vi "Teleop.vi"(10 "Match Info":T1={"Autonomous Elapsed Seconds"=0.0, "TeleOp Elapsed Seconds"=0.0, "Disabled Elapsed Seconds"=0.0, "Visited Autonomous"=FALSE, "Visited TeleOp"=FALSE, "Visited Disabled"=FALSE, "Autonomous Settings"={"Autonomous Style"=enum."Independent", "VI Refnum"=refnum}}, 11 "Call Context":T2) -> ()   [LabVIEW 2018]
doc: "This VI is called for each TeleOp packet received from the DS where the robot is not disabled. It is often used to read from the joysticks and update I/O or to update setpoints for timed control loops. It should complete and return within 20 milliseconds or it may miss DS packets."
uses:
  <vilib>/Rock Robotics/WPI/DriverStation/WPI_DriverStationDerivedRobotMode.ctl
  <vilib>/Rock Robotics/WPI/DriverStation/WPI_DriverStationMatch Info.ctl
  <vilib>/Rock Robotics/WPI/Solenoid/WPI_SolenoidValue.ctl
  <vilib>/Rock Robotics/WPI/Utilities/WPI_GetSetVariantRefNum.vi
  Robot Global Data.vi
  <vilib>/Rock Robotics/Network Tables/NT Write Numeric Array.vi
  <vilib>/Rock Robotics/WPI/Solenoid/WPI_SolenoidSetEnum.vi
  <vilib>/Rock Robotics/Network Tables/NT Write Number.vi
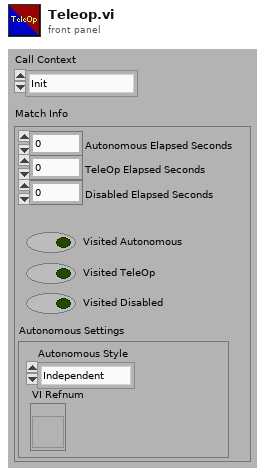
[diagram p1: front panel]
types:
  T1 = typedef "WPI_DriverStationMatch Info.ctl" = cluster{"Autonomous Elapsed Seconds":dbl, "TeleOp Elapsed Seconds":dbl, "Disabled Elapsed Seconds":dbl, "Visited Autonomous":bool, "Visited TeleOp":bool, "Visited Disabled":bool, "Autonomous Settings":cluster{"Autonomous Style":enum16{"Iterative", "Independent"}, "VI Refnum":refnum<vi>}}
  T2 = typedef "WPI_DriverStationDerivedRobotMode.ctl" = enum16{"Init", "Execute", "Stop"}
  T3 = typedef "WPI_SolenoidDevRef.ctl" = cluster{"DevStatus":errorcluster, "Pneumatics Control Module":u8, "Forward Solenoid Channel":T4, "Reverse Solenoid Channel":T4}
  T4 = typedef "WPI_SolenoidChannel.ctl" = enum8{"Solenoid 0", "Solenoid 1", "Solenoid 2", "Solenoid 3", "Solenoid 4", "Solenoid 5", "Solenoid 6", "Solenoid 7", "Invalid"}
  T5 = typedef "WPI_MotorControlDeviceRef.ctl" = cluster{"DeviceStatus":errorcluster, "Type":T6, "PWM":cluster{"PWM Channel":T7, "DeadBand":T8}, "CAN":cluster{"Device Number":u8, "SetOutput VI Ref":variant, "GetOutput VI Ref":variant, "Enable VI Ref":variant, "Disable VI Ref":variant, "Data":variant}, "Invert":bool, "DIO PWM":cluster{"PWM \"Enable\" Channel":T7, "DIOChannel":T9, "PWM Rate":dbl}}
  T6 = typedef "WPI_MotorControlType.ctl" = enum16{"PWM", "CAN", "DIO PWM"}
  T7 = typedef "FPGA_DIOPWMChannel.ctl" = enum8{"PWM 0", "PWM 1", "PWM 2", "PWM 3", "PWM 4", "PWM 5", "PWM 6", "PWM 7", "PWM 8", "PWM 9", "PWM MXP 0", "PWM MXP 1", "PWM MXP 2", "PWM MXP 3", "PWM MXP 4", "PWM MXP 5", "PWM MXP 6", "PWM MXP 7", "PWM MXP 8", "PWM MXP 9", "Invalid"}
  T8 = typedef "WPI_PWMDeadband.ctl" = cluster{"Name":string, "maxPositivePwm":i32, "minPositivePwm":i32, "centerPwm":i32, "maxNegativePwm":i32, "minNegativePwm":i32, "angularRange":u16}
  T9 = typedef "FPGA_DIOChannel.ctl" = enum8{"DIO 0", "DIO 1", "DIO 2", "DIO 3", "DIO 4", "DIO 5", "DIO 6", "DIO 7", "DIO 8", "DIO 9", "DIO MXP 0", "DIO MXP 1", "DIO MXP 2", "DIO MXP 3", "DIO MXP 4", "DIO MXP 5", "DIO MXP 6", "DIO MXP 7", "DIO MXP 8", "DIO MXP 9", "DIO MXP 10", "DIO MXP 11", "DIO MXP 12", "DIO MXP 13", "DIO MXP 14", "DIO MXP 15", "SPI Port CS1", "SPI Port CS2", "SPI Port CS3", "SPI Port MISO", "SPI Port MOSI", "Invalid"}
  T10 = typedef "WPI_SolenoidValue.ctl" = enum16{"Off", "On", "Forward", "Reverse"}
  T11 = typedef "WPI_RobotDriveDevRef.ctl" = cluster{"DevStatus":errorcluster, "Motors[]":T5[], "Square Inputs":bool, "Max Output":dbl}
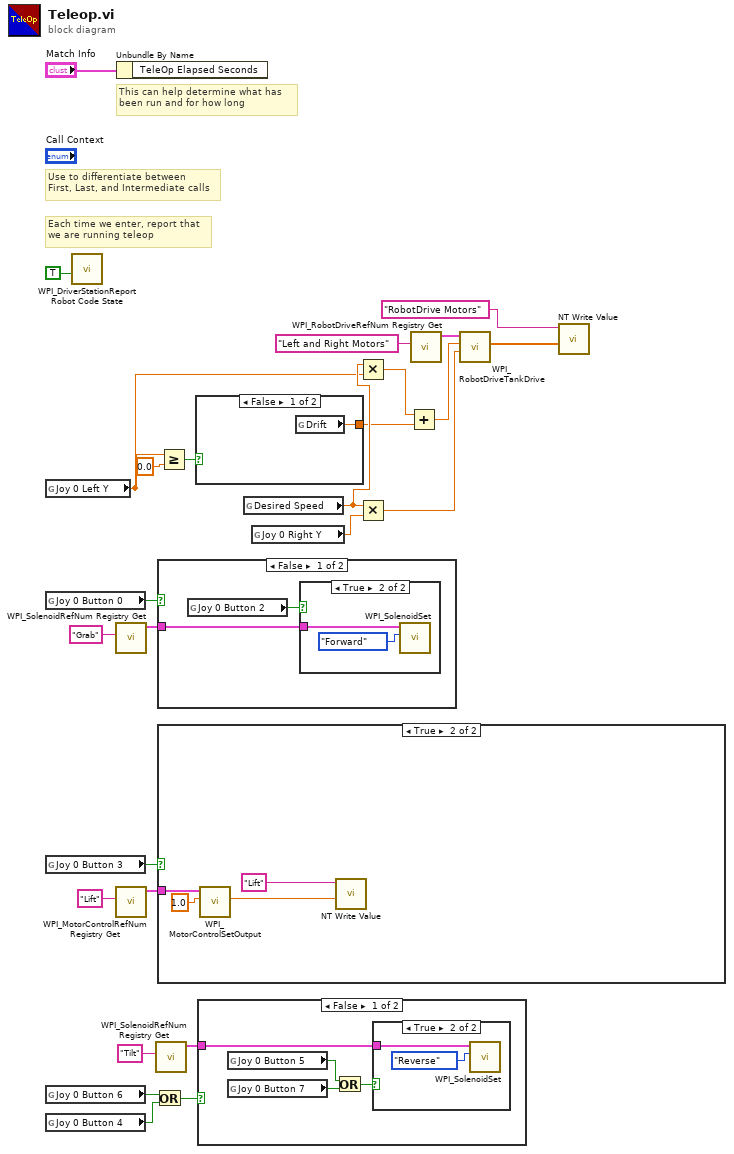
[diagram p0: block diagram]
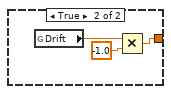
[diagram p2: hidden frame]
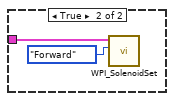
[diagram p4: hidden frame]
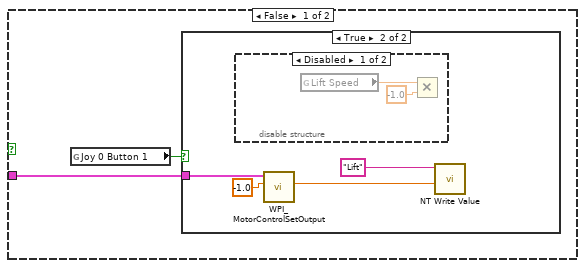
[diagram p5: hidden frame]
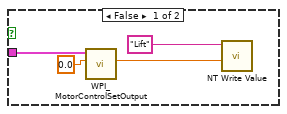
[diagram p6: hidden frame]
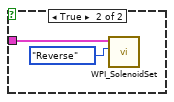
[diagram p9: hidden frame]
diagram:
  # "Each time we enter, report that\nwe are running teleop"
  # "Use to differentiate between\nFirst, Last, and Intermediate calls"
  # "This can help determine what has\nbeen run and for how long"
  n1 = global read "Robot Global Data.vi" "Joy 0 Left Y"() -> (w3:dbl)
  n2 = global read "Robot Global Data.vi" "Joy 0 Button 0"() -> (w13:bool)
  n3 = global read "Robot Global Data.vi" "Joy 0 Button 3"() -> (w11:bool)
  n4 = global read "Robot Global Data.vi" "Joy 0 Button 6"() -> (w8:bool)
  n5 = global read "Robot Global Data.vi" "Joy 0 Button 4"() -> (w9:bool)
  n6 = call <vilib>:"WPI_DriverStationReport Robot Code State.vi"("TeleOp"=TRUE ("Autonomous")) -> ()  [unwired: 10 in, 1 out]
  n7 = call <vilib>:"WPI_SolenoidRefNum Registry Get.vi"("refnum name"="Grab") -> ("SolenoidDevRef"=w14:T3)  [unwired: 9 in, 1 out]
  n8 = call <vilib>:"WPI_MotorControlRefNum Registry Get.vi"("refnum name"="Lift") -> ("MotorControlDevRef"=w10:T5)  [unwired: 9 in, 1 out]
  n9 = Unbundle By Name("Match Info") -> ()  [unwired: 1 out]
  n10 = Or(x=w8, y=w9) -> (x .or. y?=w7:bool)
  n11 = call <vilib>:"WPI_SolenoidRefNum Registry Get.vi"("refnum name"="Tilt") -> ("SolenoidDevRef"=w5:T3)  [unwired: 9 in, 1 out]
  n12 = case shown="False" w13 {
    tunnel: w14 -> [w27 w32]
    frame False {
      n13 = global read "Robot Global Data.vi" "Joy 0 Button 2"() -> (w28:bool)
      n14 = case shown="True" w28 {
        tunnel: w27 -> [_ w29]
        frame False {
        }
        frame True {
          n15 = call-poly <vilib>:"WPI_SolenoidSet.vi"("Value"=WPI_SolenoidValue."Forward", "SolenoidDevRef"=w29) -> ()  [unwired: 8 in, 2 out]
        }
      }
    }
    frame True {
      n16 = call-poly <vilib>:"WPI_SolenoidSet.vi"("Value"=WPI_SolenoidValue."Reverse", "SolenoidDevRef"=w32) -> ()  [unwired: 8 in, 2 out]
    }
  }
  n17 = case shown="True" w11 {
    tunnel: w10 -> [w33 w46]
    frame False {
      n18 = global read "Robot Global Data.vi" "Joy 0 Button 1"() -> (w34:bool)
      n19 = case shown="True" w34 {
        tunnel: w33 -> [w35 w40]
        frame False {
          n20 = call <vilib>:"WPI_MotorControlSetOutput.vi"("Output"=0.0, "MotorControlDevRef"=w35) -> ("Motor Output"=w37:dbl)  [unwired: 7 in, 2 out]
          n21 = call-poly <vilib>:"NT Write Value.vi"("Numeric"=w37, "Name"="Lift") -> ()  [unwired: 9 in, 1 out]
        }
        frame True {
          n22 = disable-structure shown="Disabled" {
            frame Disabled {
              n23 = global read "Robot Global Data.vi" "Lift Speed"() -> (w44:dbl)
              n24 = Multiply(x=w44, y=-1.0) -> ()  [unwired: 1 out]
            }
            frame Enabled {
            }
          }
          n25 = call <vilib>:"WPI_MotorControlSetOutput.vi"("Output"=-1.0, "MotorControlDevRef"=w40) -> ("Motor Output"=w41:dbl)  [unwired: 7 in, 2 out]
          n26 = call-poly <vilib>:"NT Write Value.vi"("Numeric"=w41, "Name"="Lift") -> ()  [unwired: 9 in, 1 out]
        }
      }
    }
    frame True {
      n27 = call <vilib>:"WPI_MotorControlSetOutput.vi"("Output"=1.0, "MotorControlDevRef"=w46) -> ("Motor Output"=w47:dbl)  [unwired: 7 in, 2 out]
      n28 = call-poly <vilib>:"NT Write Value.vi"("Numeric"=w47, "Name"="Lift") -> ()  [unwired: 9 in, 1 out]
    }
  }
  n29 = Greater Or Equal?(x=w3, y=0.0) -> (x >= y?=w4:bool)
  n30 = case shown="False" w4 {
    tunnel: [w49 w50] -> w1
    frame False {
      n31 = global read "Robot Global Data.vi" "Drift"() -> (w49:dbl)
    }
    frame True {
      n32 = global read "Robot Global Data.vi" "Drift"() -> (w52:dbl)
      n33 = Multiply(x=w52, y=-1.0) -> (x*y=w50:dbl)
    }
  }
  n34 = case shown="False" w7 {
    tunnel: w5 -> [w53 w59]
    frame False {
      n35 = global read "Robot Global Data.vi" "Joy 0 Button 5"() -> (w55:bool)
      n36 = global read "Robot Global Data.vi" "Joy 0 Button 7"() -> (w56:bool)
      n37 = Or(x=w55, y=w56) -> (x .or. y?=w54:bool)
      n38 = case shown="True" w54 {
        tunnel: w53 -> [_ w57]
        frame False {
        }
        frame True {
          n39 = call-poly <vilib>:"WPI_SolenoidSet.vi"("Value"=WPI_SolenoidValue."Reverse", "SolenoidDevRef"=w57) -> ()  [unwired: 8 in, 2 out]
        }
      }
    }
    frame True {
      n40 = call-poly <vilib>:"WPI_SolenoidSet.vi"("Value"=WPI_SolenoidValue."Forward", "SolenoidDevRef"=w59) -> ()  [unwired: 8 in, 2 out]
    }
  }
  n41 = global read "Robot Global Data.vi" "Desired Speed"() -> (w24:dbl)
  n42 = global read "Robot Global Data.vi" "Joy 0 Right Y"() -> (w23:dbl)
  n43 = Multiply(x=w24, y=w3) -> (x*y=w22:dbl)
  n44 = Multiply(x=w24, y=w23) -> (x*y=w16:dbl)
  n45 = Add(x=w22, y=w1) -> (x+y=w17:dbl)
  n46 = call <vilib>:"WPI_RobotDriveRefNum Registry Get.vi"("refnum name"="Left and Right Motors") -> ("RobotDriveDevRef"=w18:T11)  [unwired: 1 in, 9 out]
  n47 = call <vilib>:"WPI_RobotDriveTankDrive.vi"("Right axis value"=w16, "Left axis value"=w17, "RobotDriveDevRef"=w18) -> ("Motor Values"=w19:dbl[])  [unwired: 6 in, 2 out]
  n48 = call-poly <vilib>:"NT Write Value.vi"("Numeric Array"=w19, "Name"="RobotDrive Motors") -> ()  [unwired: 9 in, 1 out]
